vi "User Get Current Logins.vi"(8 "error in (no error)":errorcluster, 10 "Current User (none)":T1, 11 "Connection Refnum":T2) -> (0 "error out":errorcluster, 1 "Current User Summary":string, 2 "Seats in Use":i32, 3 "dup Connection Refnum":T2, 5 "Current User has Seat?":bool)   [LabVIEW 2011]
uses:
  SI.LIB/ODBC/SQL Controls/Connection Refnum.ctl
  User Record.ctl
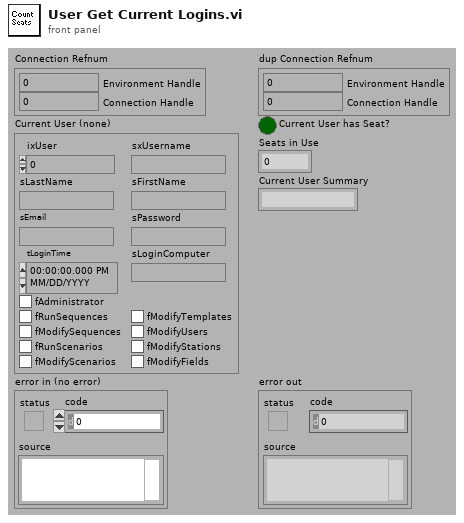
[diagram p1: front panel]
types:
  T1 = typedef "User Record.ctl" = cluster{"ixUser":i32, "sxUsername":string, "sLastName":string, "sFirstName":string, "sEmail":string, "sPassword":string, "tLoginTime":timestamp, "sLoginComputer":string, "fAdministrator":bool, "fRunSequences":bool, "fModifySequences":bool, "fRunScenarios":bool, "fModifyScenarios":bool, "fModifyTemplates":bool, "fModifyUsers":bool, "fModifyStations":bool, "fModifyFields":bool}
  T2 = typedef "Connection Refnum.ctl" = cluster{"Environment Handle":i32, "Connection Handle":i32}
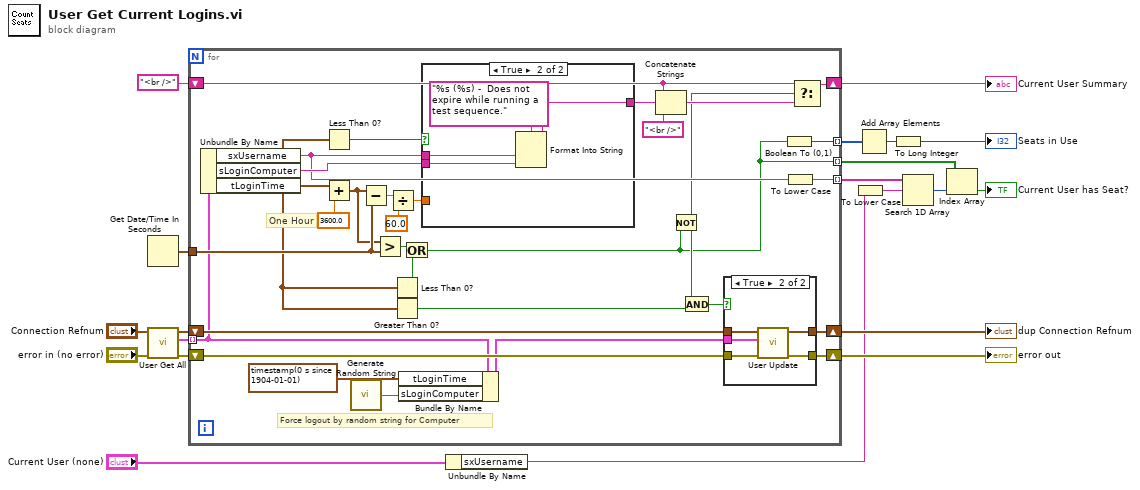
[diagram p0: block diagram]
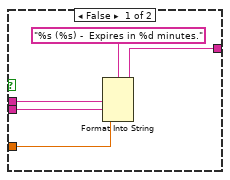
[diagram p2: hidden frame]
diagram:
  n1 = Get Date/Time In Seconds() -> (seconds since 1Jan1904=w11:timestamp)
  n2 = call "User Get All.vi"("error in (no error)"="error in (no error)", "Connection Refnum"="Connection Refnum") -> ("error out"=w17:errorcluster, "User Records"=w20:T1[], "Connection Refnum"=w12:T2)  [unwired: 2 in, 5 out]
  n3 = for {
    tunnel: w20 -> [w31] mode=indexing
    tunnel: w11 -> [w41]
    tunnel: [w50] -> w19 mode=indexing
    shift-right: [w46] -> w8
    shift-left: w17 -> [w47]
    shift-right: [w45] -> w1
    shift-left: "<br />" -> [w28]
    tunnel: [w33] -> w14 mode=indexing
    tunnel: [w23] -> w15 mode=indexing
    shift-right: [w34] -> w6
    shift-left: w12 -> [w35]
    # "Force logout by random string for Computer"
    # "One Hour"
    n4 = Unbundle By Name(w31) -> ("sxUsername"=w36:string, "sLoginComputer"=w43:string, "tLoginTime"=w22:timestamp)
    n5 = Less Than 0?(x=w22) -> (x < 0?=w25:bool)
    n6 = Add(x=w22, y=3600.0) -> (x+y=w40:timestamp)
    n7 = call "Generate Random String.vi"() -> ("Output String"=w29:string)  [unwired: 1 in, 4 out]
    n8 = Subtract(x=w40, y=w41) -> (x-y=w39:dbl)
    n9 = Greater?(x=w40, y=w41) -> (0:w24:bool)
    n10 = Divide(x=w39, y=60.0) -> (x/y=w37:dbl)
    n11 = Less Than 0?(x=w22) -> (x < 0?=w21:bool)
    n12 = Greater Than 0?(x=w22) -> (x > 0?=w49:bool)
    n13 = Bundle By Name(cluster=w31, "tLoginTime"=timestamp(0 s since 1904-01-01), "sLoginComputer"=w29) -> (w30:T1)
    n14 = Or(x=w24, y=w21) -> (x .or. y?=w23:bool)
    n15 = case shown="True" w25 {
      tunnel: w43 -> [w55 w59]
      tunnel: [w54 w58] -> w42
      tunnel: w37 -> [w53 _]
      tunnel: w36 -> [w52 w57]
      frame False {
        n16 = Format Into String(format string="%s (%s) -  Expires in %d minutes.", w52, w55, w53) -> (resulting string=w54:string)  [unwired: 2 in, 1 out]
      }
      frame True {
        n17 = Format Into String(format string="%s (%s) -  Does not expire while running a test sequence.", w57, w59) -> (resulting string=w58:string)  [unwired: 2 in, 1 out]
      }
    }
    n18 = Concatenate Strings(w28, w42, "<br />") -> (w27:string)
    n19 = Not(x=w23) -> (.not. x?=w26:bool)
    n20 = And(x=w26, y=w49) -> (x .and. y?=w48:bool)
    n21 = case shown="True" w48 {
      tunnel: w47 -> [w62 w67]
      tunnel: w30 -> [_ w63]
      tunnel: [w62 w66] -> w46
      tunnel: w35 -> [w61 w65]
      tunnel: [w61 w64] -> w34
      frame False {
      }
      frame True {
        n22 = call "User Update.vi"("error in (no error)"=w67, "User Record"=w63, "Connection Refnum"=w65) -> ("error out"=w66:errorcluster, "dup Connection Refnum"=w64:T2)  [unwired: 7 out]
      }
    }
    n23 = Boolean To (0,1)(Boolean=w23) -> (0, 1=w50:i16)
    n24 = To Lower Case(string=w36) -> (all lower case string=w33:string)
    n25 = Select(t=w28, s=w26, f=w27) -> (s? t:f=w45:string)
  }
  "error out" <- w8
  "dup Connection Refnum" <- w6
  "Current User Summary" <- w1
  n26 = Unbundle By Name("Current User (none)") -> ("sxUsername"=w4:string)
  n27 = To Lower Case(string=w4) -> (all lower case string=w10:string)
  n28 = Add Array Elements(numeric array=w19) -> (sum=w18:i16)
  n29 = To Long Integer(number=w18) -> (32bit integer=→"Seats in Use":i32)
  n30 = Search 1D Array(1D array=w14, element=w10) -> (index of element=w13:i32)  [unwired: 1 out]
  n31 = Index Array(array=w15, index=w13) -> (element=→"Current User has Seat?":bool)
